vi "Get elapsed time.vi"(8 "error in (no error)":errorcluster, 11 "Timer name":string) -> (0 "error out":errorcluster, 1 "Elapsed time (minutes)":dbl, 2 "Elapsed time (s)":dbl, 3 "Elapsed time (ms)":u32)   [LabVIEW 2021, in "Named Timers.lvlib"]
uses:
  Named Timers.lvlib
  Timer global variable.vi
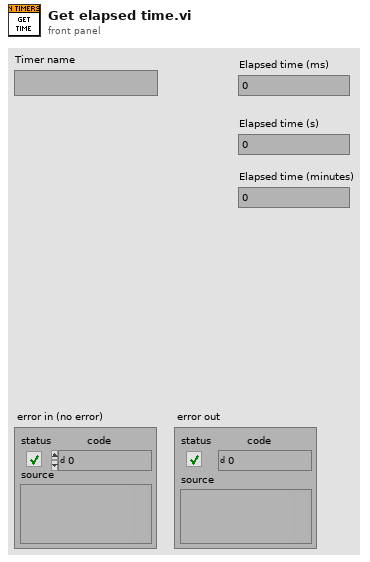
[diagram p1: front panel]
types:
  T1 = typedef "Named Timers.lvlib/Timer Cluster.ctl" = cluster{"Name":string, "Start time (ms)":u32}
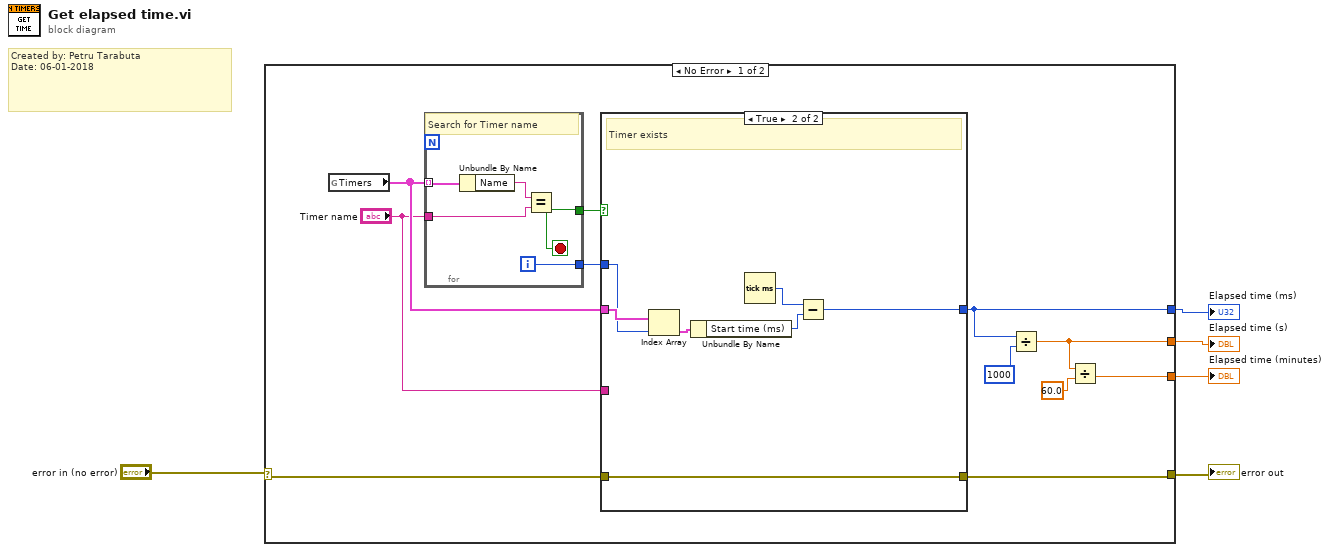
[diagram p0: block diagram]
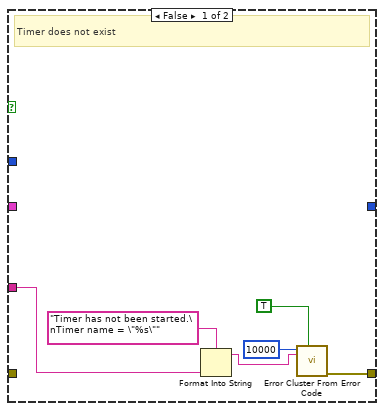
[diagram p2: hidden frame]
diagram:
  # "Created by: Petru Tarabuta\nDate: 06-01-2018"
  n1 = case shown="No Error" "error in (no error)" {
    selector: "error in (no error)" -> [w11 w35]
    tunnel: [w12 w35] -> w4
    tunnel: [w10 _] -> w3
    tunnel: [w7 _] -> w2
    tunnel: [w6 _] -> w1
    frame No Error {
      n2 = global read "Timer global variable.vi" "Timers"() -> (w15:T1[])
      n3 = for {
        tunnel: w15 -> [w34] mode=indexing
        tunnel: "Timer name" -> [w32]
        tunnel: [w31] -> w16
        tunnel: [w30] -> w13
        i -> [w30]
        stop <- w31 stop-if-true
        # "Search for Timer name"
        n4 = Unbundle By Name(w34) -> ("Name"=w33:string)
        n5 = Equal?(x=w33, y=w32) -> (x = y?=w31:bool)
      }
      n6 = case shown="True" w16 {
        tunnel: w15 -> [_ w28]
        tunnel: "Timer name" -> [w17 _]
        tunnel: w13 -> [_ w27]
        tunnel: [w22 w26] -> w12
        tunnel: w11 -> [_ w26]
        tunnel: [_ w23] -> w10
        frame False {
          # "Timer does not exist"
          n7 = Format Into String(format string="Timer has not been started.\nTimer name = \"%s\"" ("error message (\"\")"), w17) -> (resulting string=w18:string)  [unwired: 2 in, 1 out]
          n8 = call <vilib>:"Error Cluster From Error Code.vi"("show call chain? (False)"=TRUE, "error message (\"\")"=w18, "error code (0)"=10000) -> ("error out"=w22:errorcluster)  [unwired: 6 in]
        }
        frame True {
          # "Timer exists"
          n9 = Index Array(array=w28, index=w27) -> (element=w29:T1)
          n10 = Unbundle By Name(w29) -> ("Start time (ms)"=w25:u32)
          n11 = Tick Count (ms)() -> (millisecond timer value=w24:u32)
          n12 = Subtract(x=w24, y=w25) -> (x-y=w23:u32)
        }
      }
      n13 = Divide(x=w10, y=u32 1000) -> (x/y=w7:dbl)
      n14 = Divide(x=w7, y=60.0) -> (x/y=w6:dbl)
    }
    frame Error {
    }
  }
  "error out" <- w4
  "Elapsed time (ms)" <- w3
  "Elapsed time (s)" <- w2
  "Elapsed time (minutes)" <- w1
